vi "VolumeAndTimeSamplesvi.vi"() -> ()   [LabVIEW 2013]
panel:
  in  "VolumeAndTimeSamples":T1
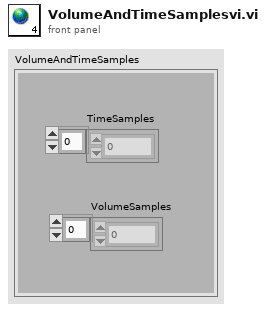
[diagram p1: front panel]
types:
  T1 = cluster{"TimeSamples":dbl[], "VolumeSamples":dbl[]}
diagram:
